vi "Фиксироание всех параметров (SubVI).vi"(1 "Параметры всех мишеней":T6, 3 "Видимость мишеней":T3, 4 "error in":errorcluster, 5 "полож. красной точки лазера":T2, 6 "полож. текущ. инф.":T2, 8 "Знаки Dx всех мишеней":T1={"Знак перех. dX М1"=1, "Знак перех. dX М2"=0, "Знак перех. dX М3"=0, "Знак перех. dX М4"=0, "Знак перех. dX М5"=0, "Знак перех. dX М6"=0, "Знак перех. dX М7"=0, "Знак перех. dX М8"=0, "Знак перех. dX М9"=0, "Знак перех. dX М10"=0}, 9 "Текущ. положение лазера на мишенях 1 - 5":T4, 10 "текущий id мишени":u16=1, 12 "Выстрелов осталось по всем мишеням":T5, 13 "Текущ. положение лазера на мишенях 6 - 10":T4) -> (23 "Строка параметров мишеней для сохранения":string, 27 "error out":errorcluster)   [LabVIEW 2013]
doc: "Фиксирование всех параметров системы для сохранения текузей конфигурации"
uses:
  <vilib>/Utility/miscctls.llb/LVPositionTypeDef.ctl
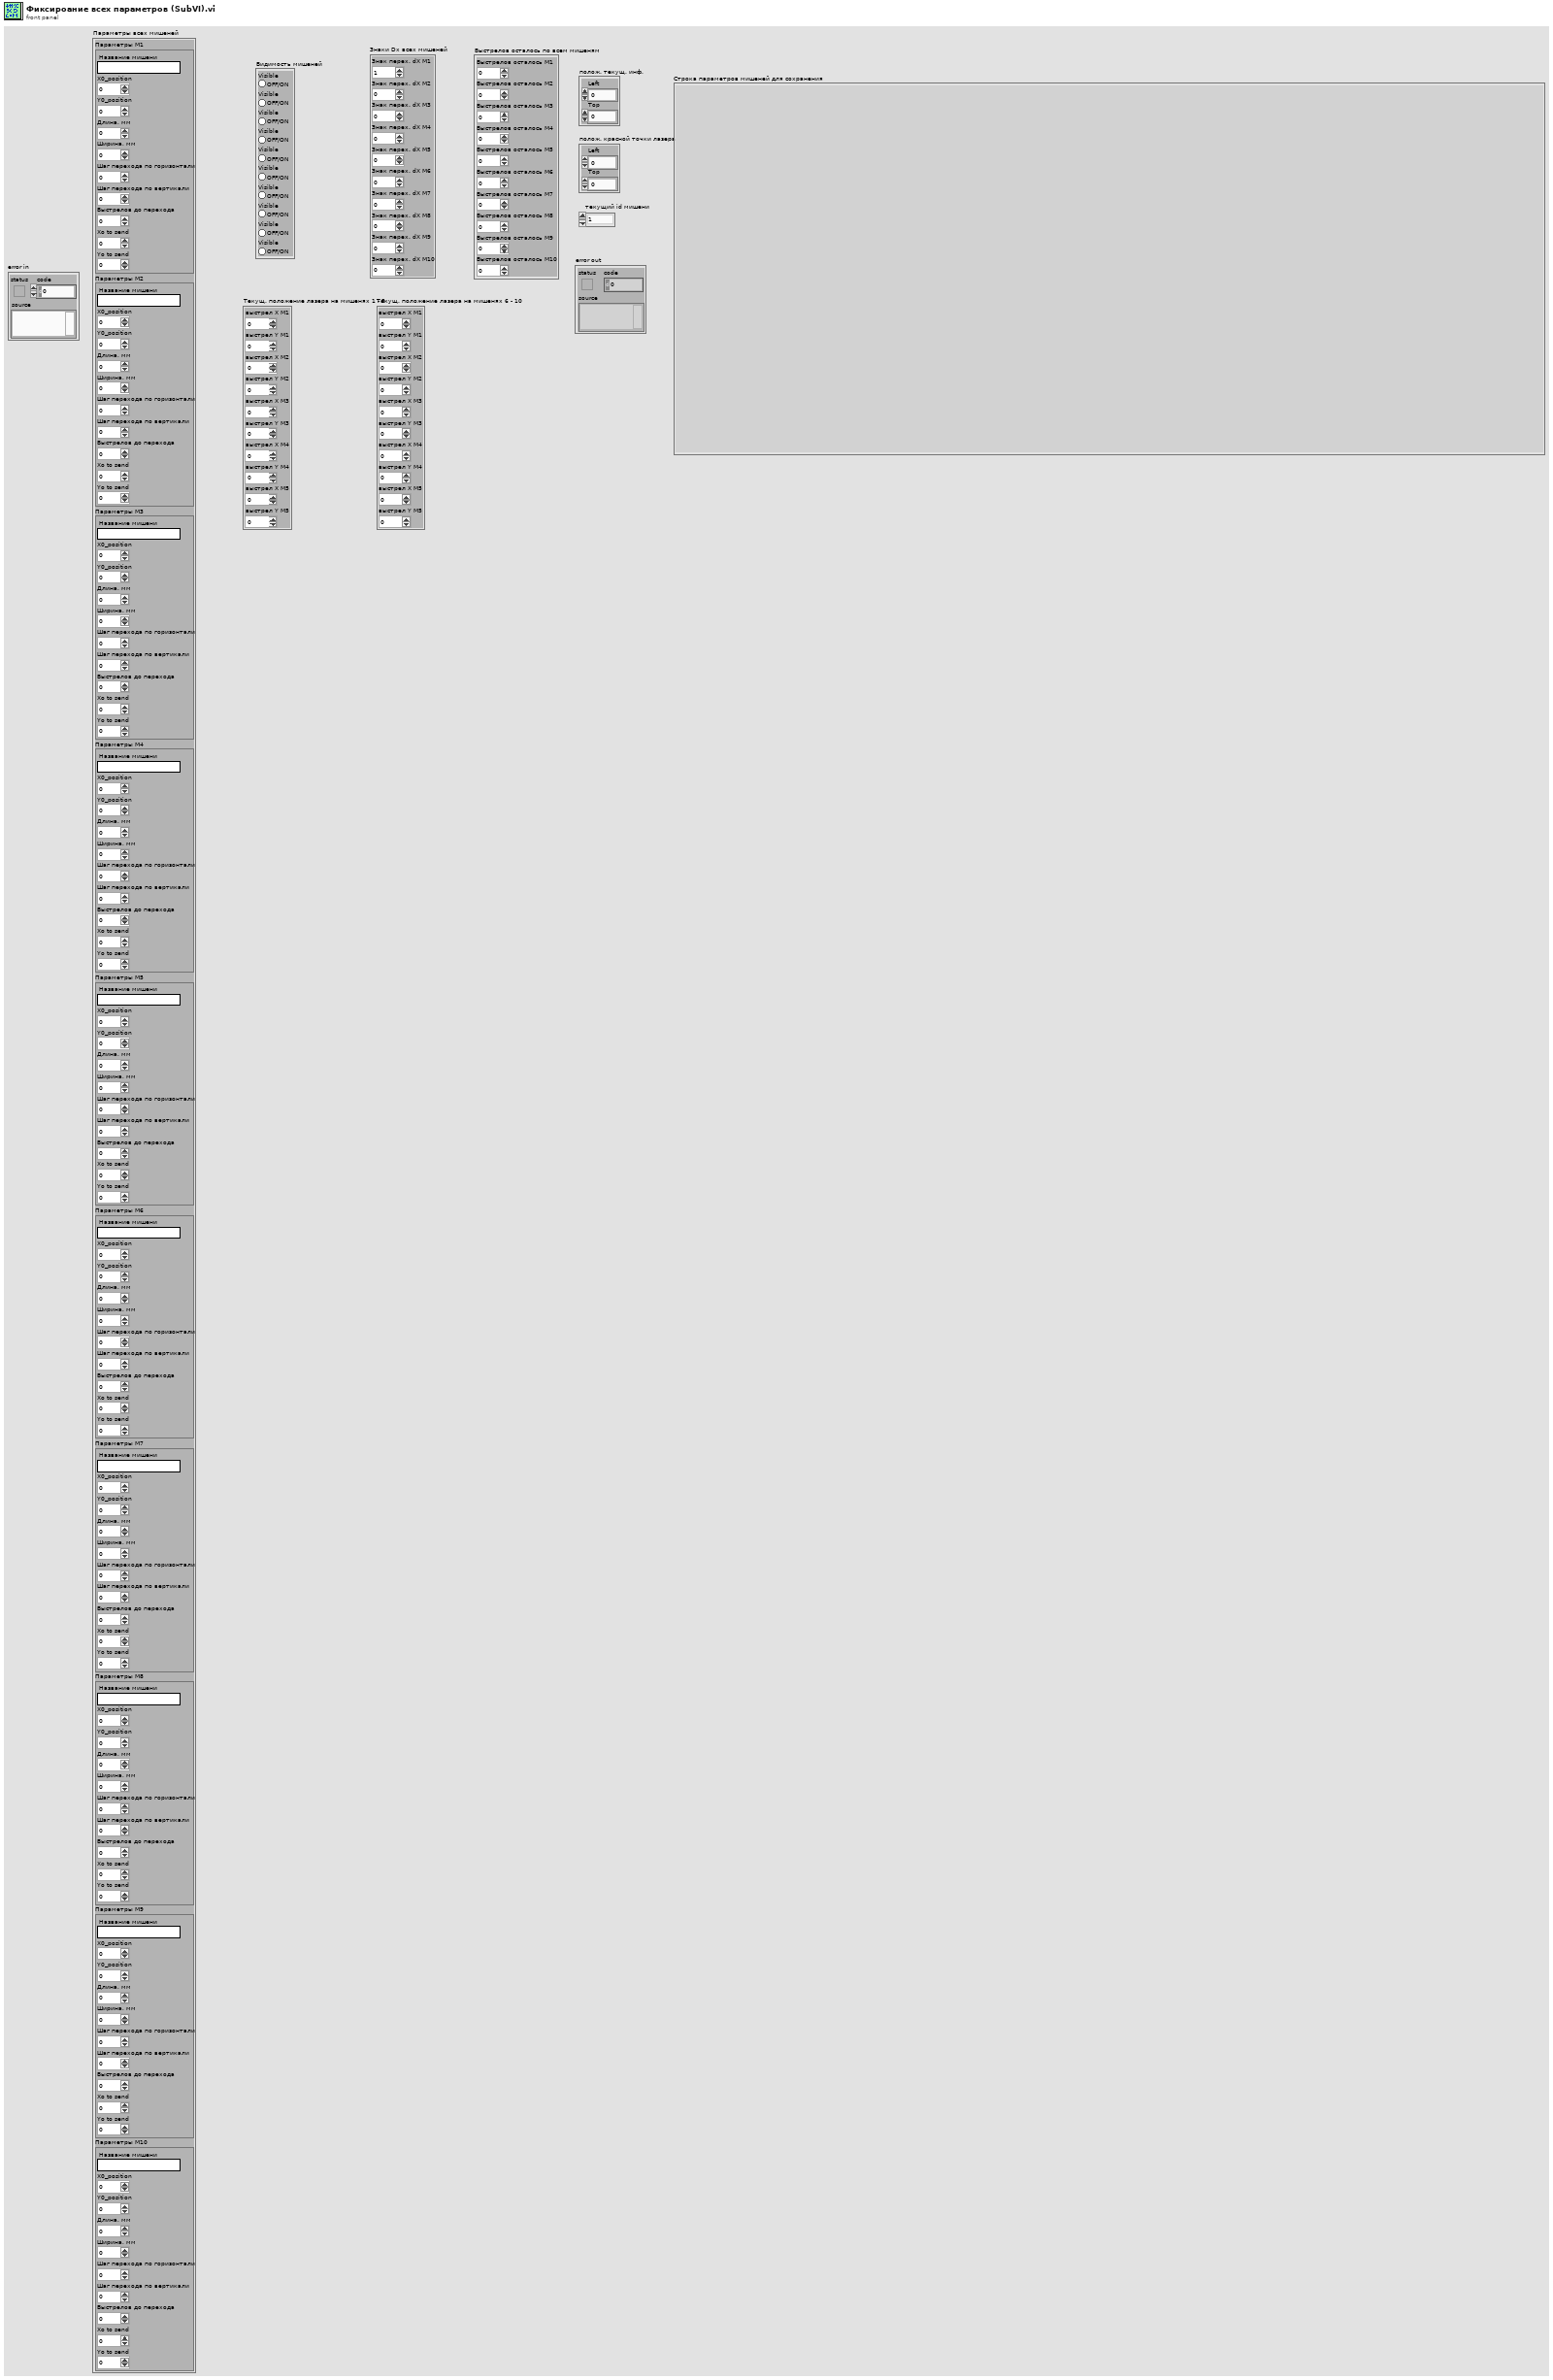
[diagram p1: front panel]
types:
  T1 = cluster{"Знак перех. dX М1":i8, "Знак перех. dX М2":i8, "Знак перех. dX М3":i8, "Знак перех. dX М4":i8, "Знак перех. dX М5":i8, "Знак перех. dX М6":i8, "Знак перех. dX М7":i8, "Знак перех. dX М8":i8, "Знак перех. dX М9":i8, "Знак перех. dX М10":i8}
  T2 = typedef "LVPositionTypeDef.ctl" = cluster{"Left":i32, "Top":i32}
  T3 = cluster{"Visible":bool, "Visible":bool, "Visible":bool, "Visible":bool, "Visible":bool, "Visible":bool, "Visible":bool, "Visible":bool, "Visible":bool, "Visible":bool}
  T4 = cluster{"выстрел X М1":u16, "выстрел Y М1":u16, "выстрел X М2":u16, "выстрел Y М2":u16, "выстрел X М3":u16, "выстрел Y М3":u16, "выстрел X М4":u16, "выстрел Y М4":u16, "выстрел X М5":u16, "выстрел Y М5":u16}
  T5 = cluster{"Выстрелов осталось M1 ":u16, "Выстрелов осталось M2":u16, "Выстрелов осталось M3":u16, "Выстрелов осталось M4":u16, "Выстрелов осталось M5":u16, "Выстрелов осталось M6":u16, "Выстрелов осталось M7":u16, "Выстрелов осталось M8":u16, "Выстрелов осталось M9":u16, "Выстрелов осталось M10":u16}
  T6 = cluster{"Параметры М1":cluster{"Название мишени":string, "Х0_position":u16, "Y0_position":u16, "Длина, мм":u16, "Ширина, мм":u16, "Шаг перехода по горизонтали":dbl, "Шаг перехода по вертикали":dbl, "Выстрелов до перехода":u16, "Xo to send ":u16, "Yo to send":u16}, "Параметры М2":cluster{"Название мишени":string, "Х0_position":u16, "Y0_position":u16, "Длина, мм":u16, "Ширина, мм":u16, "Шаг перехода по горизонтали":dbl, "Шаг перехода по вертикали":dbl, "Выстрелов до перехода":u16, "Xo to send ":u16, "Yo to send":u16}, "Параметры М3":cluster{"Название мишени":string, "Х0_position":u16, "Y0_position":u16, "Длина, мм":u16, "Ширина, мм":u16, "Шаг перехода по горизонтали":dbl, "Шаг перехода по вертикали":dbl, "Выстрелов до перехода":u16, "Xo to send ":u16, "Yo to send":u16}, "Параметры М4":cluster{"Название мишени":string, "Х0_position":u16, "Y0_position":u16, "Длина, мм":u16, "Ширина, мм":u16, "Шаг перехода по горизонтали":dbl, "Шаг перехода по вертикали":dbl, "Выстрелов до перехода":u16, "Xo to send ":u16, "Yo to send":u16}, "Параметры М5":cluster{"Название мишени":string, "Х0_position":u16, "Y0_position":u16, "Длина, мм":u16, "Ширина, мм":u16, "Шаг перехода по горизонтали":dbl, "Шаг перехода по вертикали":dbl, "Выстрелов до перехода":u16, "Xo to send ":u16, "Yo to send":u16}, "Параметры М6":cluster{"Название мишени":string, "Х0_position":u16, "Y0_position":u16, "Длина, мм":u16, "Ширина, мм":u16, "Шаг перехода по горизонтали":dbl, "Шаг перехода по вертикали":dbl, "Выстрелов до перехода":u16, "Xo to send ":u16, "Yo to send":u16}, "Параметры М7":cluster{"Название мишени":string, "Х0_position":u16, "Y0_position":u16, "Длина, мм":u16, "Ширина, мм":u16, "Шаг перехода по горизонтали":dbl, "Шаг перехода по вертикали":dbl, "Выстрелов до перехода":u16, "Xo to send ":u16, "Yo to send":u16}, "Параметры М8":cluster{"Название мишени":string, "Х0_position":u16, "Y0_position":u16, "Длина, мм":u16, "Ширина, мм":u16, "Шаг перехода по горизонтали":dbl, "Шаг перехода по вертикали":dbl, "Выстрелов до перехода":u16, "Xo to send ":u16, "Yo to send":u16}, "Параметры М9":cluster{"Название мишени":string, "Х0_position":u16, "Y0_position":u16, "Длина, мм":u16, "Ширина, мм":u16, "Шаг перехода по горизонтали":dbl, "Шаг перехода по вертикали":dbl, "Выстрелов до перехода":u16, "Xo to send ":u16, "Yo to send":u16}, "Параметры М10":cluster{"Название мишени":string, "Х0_position":u16, "Y0_position":u16, "Длина, мм":u16, "Ширина, мм":u16, "Шаг перехода по горизонтали":dbl, "Шаг перехода по вертикали":dbl, "Выстрелов до перехода":u16, "Xo to send ":u16, "Yo to send":u16}}
  T7 = cluster{"Название мишени":string, "Х0_position":u16, "Y0_position":u16, "Длина, мм":u16, "Ширина, мм":u16, "Шаг перехода по горизонтали":dbl, "Шаг перехода по вертикали":dbl, "Выстрелов до перехода":u16, "Xo to send ":u16, "Yo to send":u16}
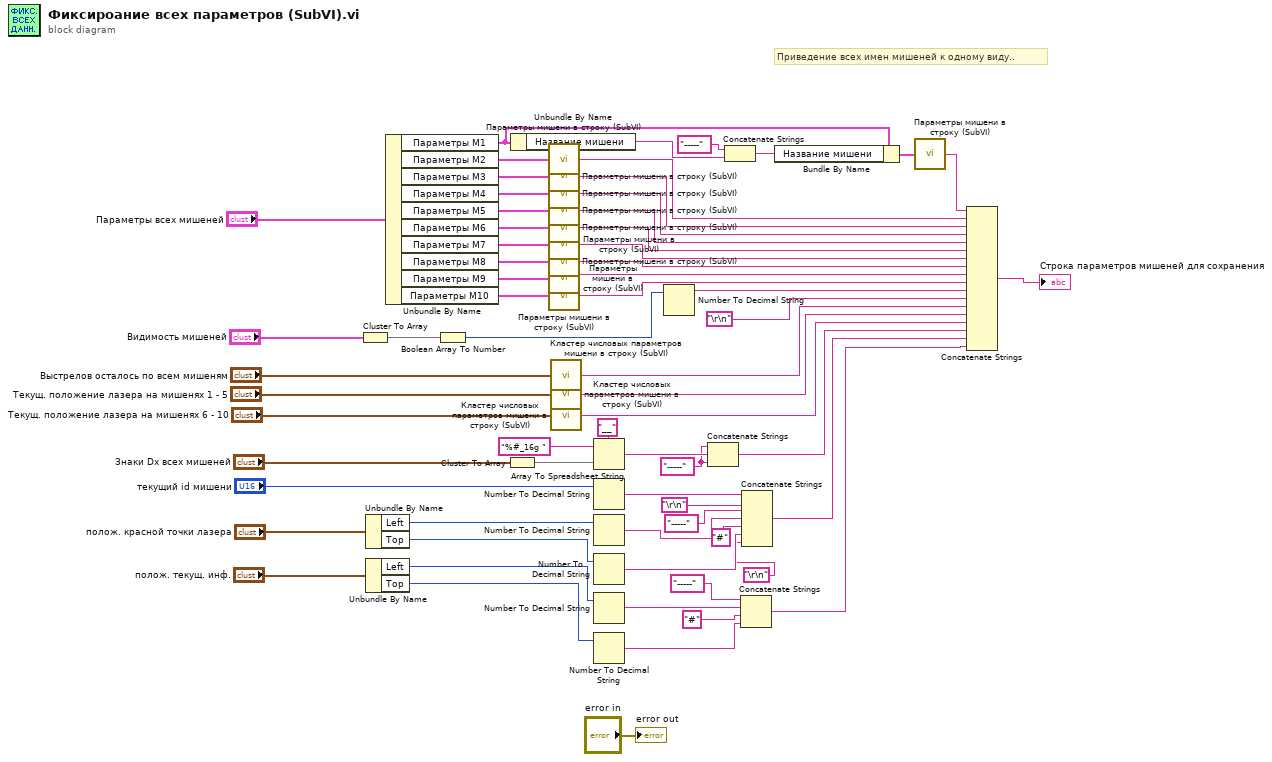
[diagram p0: block diagram]
diagram:
  w20 = "-----" ("string")
  # "Приведение всех имен мишеней к одному виду.."
  n1 = Cluster To Array(cluster="Видимость мишеней") -> (array=w62:bool[])
  n2 = Unbundle By Name("полож. красной точки лазера") -> ("Left"=w17:i32, "Top"=w16:i32)
  n3 = Unbundle By Name("полож. текущ. инф.") -> ("Left"=w15:i32, "Top"=w14:i32)
  n4 = Unbundle By Name("Параметры всех мишеней") -> ("Параметры М1"=w37:T7, "Параметры М2"=w60:T7, "Параметры М3"=w59:T7, "Параметры М4"=w58:T7, "Параметры М5"=w57:T7, "Параметры М6"=w56:T7, "Параметры М7"=w55:T7, "Параметры М8"=w54:T7, "Параметры М9"=w53:T7, "Параметры М10"=w52:T7)
  n5 = Boolean Array To Number(Boolean array=w62) -> (number=w61:u32)
  n6 = Cluster To Array(cluster="Знаки Dx всех мишеней") -> (array=w23:i8[])
  n7 = Unbundle By Name(w37) -> ("Название мишени"=w40:string)
  n8 = call "Параметры мишени в строку (SubVI).vi"("Кластер параметров мишени"=w60) -> ("Параметры мишени строка"=w42:string)  [unwired: 2 in]
  n9 = call "Параметры мишени в строку (SubVI).vi"("Кластер параметров мишени"=w59) -> ("Параметры мишени строка"=w41:string)  [unwired: 2 in]
  n10 = call "Параметры мишени в строку (SubVI).vi"("Кластер параметров мишени"=w58) -> ("Параметры мишени строка"=w51:string)  [unwired: 2 in]
  n11 = call "Параметры мишени в строку (SubVI).vi"("Кластер параметров мишени"=w57) -> ("Параметры мишени строка"=w50:string)  [unwired: 2 in]
  n12 = call "Параметры мишени в строку (SubVI).vi"("Кластер параметров мишени"=w56) -> ("Параметры мишени строка"=w49:string)  [unwired: 2 in]
  n13 = call "Параметры мишени в строку (SubVI).vi"("Кластер параметров мишени"=w55) -> ("Параметры мишени строка"=w48:string)  [unwired: 2 in]
  n14 = call "Параметры мишени в строку (SubVI).vi"("Кластер параметров мишени"=w54) -> ("Параметры мишени строка"=w47:string)  [unwired: 2 in]
  n15 = call "Параметры мишени в строку (SubVI).vi"("Кластер параметров мишени"=w53) -> ("Параметры мишени строка"=w46:string)  [unwired: 2 in]
  n16 = call "Параметры мишени в строку (SubVI).vi"("Кластер параметров мишени"=w52) -> ("Параметры мишени строка"=w45:string)  [unwired: 2 in]
  n17 = call "Кластер числовых параметров мишени в строку (SubVI).vi"("Кластер числовых параметров мишени"="Выстрелов осталось по всем мишеням") -> ("Строка числовых парам. мишени + переход на новую сторку"=w33:string)
  n18 = call "Кластер числовых параметров мишени в строку (SubVI).vi"("Кластер числовых параметров мишени"="Текущ. положение лазера на мишенях 1 - 5") -> ("Строка числовых парам. мишени + переход на новую сторку"=w31:string)
  n19 = call "Кластер числовых параметров мишени в строку (SubVI).vi"("Кластер числовых параметров мишени"="Текущ. положение лазера на мишенях 6 - 10") -> ("Строка числовых парам. мишени + переход на новую сторку"=w29:string)
  n20 = Array To Spreadsheet String(delimiter (Tab)="__", array=w23, 3:"%#_16g " ("format string")) -> (spreadsheet string=w27:string)
  n21 = Number To Decimal String(number="текущий id мишени") -> (decimal integer string=w13:string)  [unwired: 1 in]
  n22 = Number To Decimal String(number=w17) -> (decimal integer string=w9:string)  [unwired: 1 in]
  n23 = Number To Decimal String(number=w16) -> (decimal integer string=w7:string)  [unwired: 1 in]
  n24 = Number To Decimal String(number=w15) -> (decimal integer string=w4:string)  [unwired: 1 in]
  n25 = Number To Decimal String(number=w14) -> (decimal integer string=w2:string)  [unwired: 1 in]
  n26 = Number To Decimal String(number=w61) -> (decimal integer string=w35:string)  [unwired: 1 in]
  n27 = Concatenate Strings(w20, w27, w20) -> (w22:string)
  n28 = Concatenate Strings("-----" ("string"), w40) -> (w38:string)
  n29 = Concatenate Strings("-----" ("string"), w4, "#" ("string"), w2) -> (w1:string)
  n30 = Concatenate Strings(w13, "\r\n", "-----" ("string"), w9, "#" ("string"), w7, "\r\n") -> (w12:string)
  n31 = Bundle By Name(cluster=w37, "Название мишени"=w38) -> (w36:T7)
  n32 = call "Параметры мишени в строку (SubVI).vi"("Кластер параметров мишени"=w36) -> ("Параметры мишени строка"=w43:string)  [unwired: 2 in]
  n33 = Concatenate Strings(w43, w42, w41, w51, w50, w49, w48, w47, w46, w45, w35, "\r\n", w33, w31, w29, w22, w12, w1) -> (→"Строка параметров мишеней для сохранения":string)
  "error out" <- "error in"
